vi "dfd_Compute Freq Vector from Num of Bins.vi"(11 "# freq bins (512)":i32=512) -> (3 "freq points":dbl[](array[numeric]))   [LabVIEW 2017, in "NI_DigFilterLicensed.lvlib"]
uses:
  <vilib>/addons/Digital Filter Design/NI_DigFilterLicensed.lvlib
  <vilib>/Analysis/1siggen.llb/Ramp Pattern by Samples.vi
  <vilib>/Analysis/NI_AALBase.lvlib
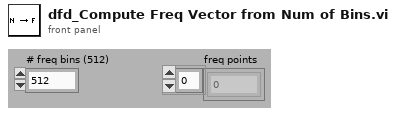
[diagram p1: front panel]
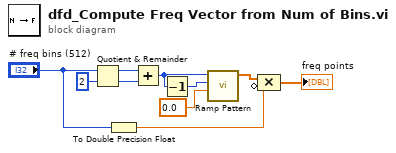
[diagram p0: block diagram]
diagram:
  n1 = Quotient & Remainder(x="# freq bins (512)", y=2) -> (x-y*floor(x/y)=w5:i32, floor(x/y)=w4:i32)
  n2 = To Double Precision Float(number="# freq bins (512)") -> (double precision float=w2:dbl)
  n3 = Add(x=w5, y=w4) -> (x+y=w3:i32)
  n4 = Decrement(x=w3) -> (x-1=w7:i32)
  n5 = call-poly <vilib>:"Ramp Pattern.vi"("start"=0.0, "end"=w7, "samples"=w3) -> ("Ramp Pattern"=w8:dbl[])  [unwired: 7 in, 1 out]
  n6 = Compound Arithmetic op=MULTIPLY(w8, invert w2) -> (→"freq points":dbl[])
